vi "parse property values into string text.vi"(0 "String in":string, 2 "Property value":variant, 5 "error in (no error)":errorcluster) -> (14 "String out":string, 19 "error out":errorcluster)   [LabVIEW 2019, in "metadata.lvclass"]
doc: "parses the property names into a string text to view the property names and parameters side by side"
uses:
  metadata.lvclass
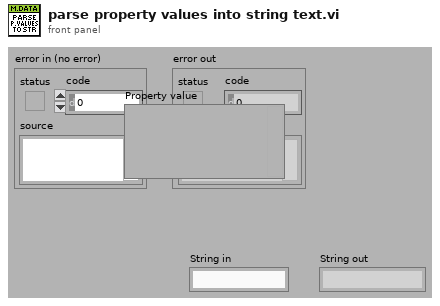
[diagram p1: front panel]
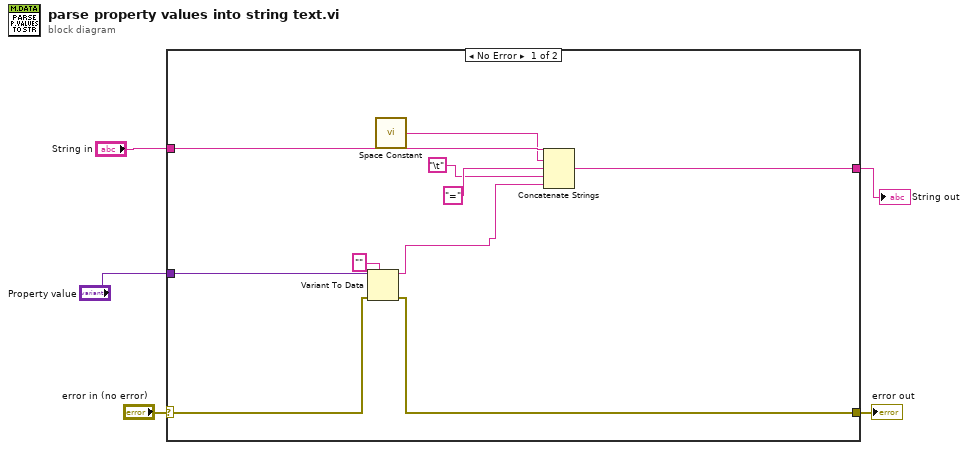
[diagram p0: block diagram]
diagram:
  n1 = case shown="No Error" "error in (no error)" {
    selector: "error in (no error)" -> [w11 w17]
    tunnel: [w10 w17] -> w4
    tunnel: [w15 w16] -> w3
    tunnel: "String in" -> [w14 w16]
    tunnel: "Property value" -> [w12 _]
    frame No Error {
      n2 = Variant To Data(error in=w11, type="" ("Property names"), Variant=w12) -> (data=w6:string, error out=w10:errorcluster)
      n3 = call <vilib>:"Space Constant.vi"() -> ("String"=w9:string)
      n4 = Concatenate Strings(w14, w9, "=" ("string"), "\t", w6) -> (w15:string)
    }
    frame Error {
    }
  }
  "error out" <- w4
  "String out" <- w3
